vi "wechatDetectCoffeeModel.vi"() -> (0 "Model":string, 1 "ProtoTxt":string)   [LabVIEW 2020]
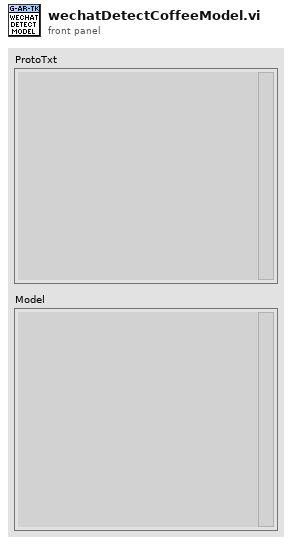
[diagram p1: front panel]
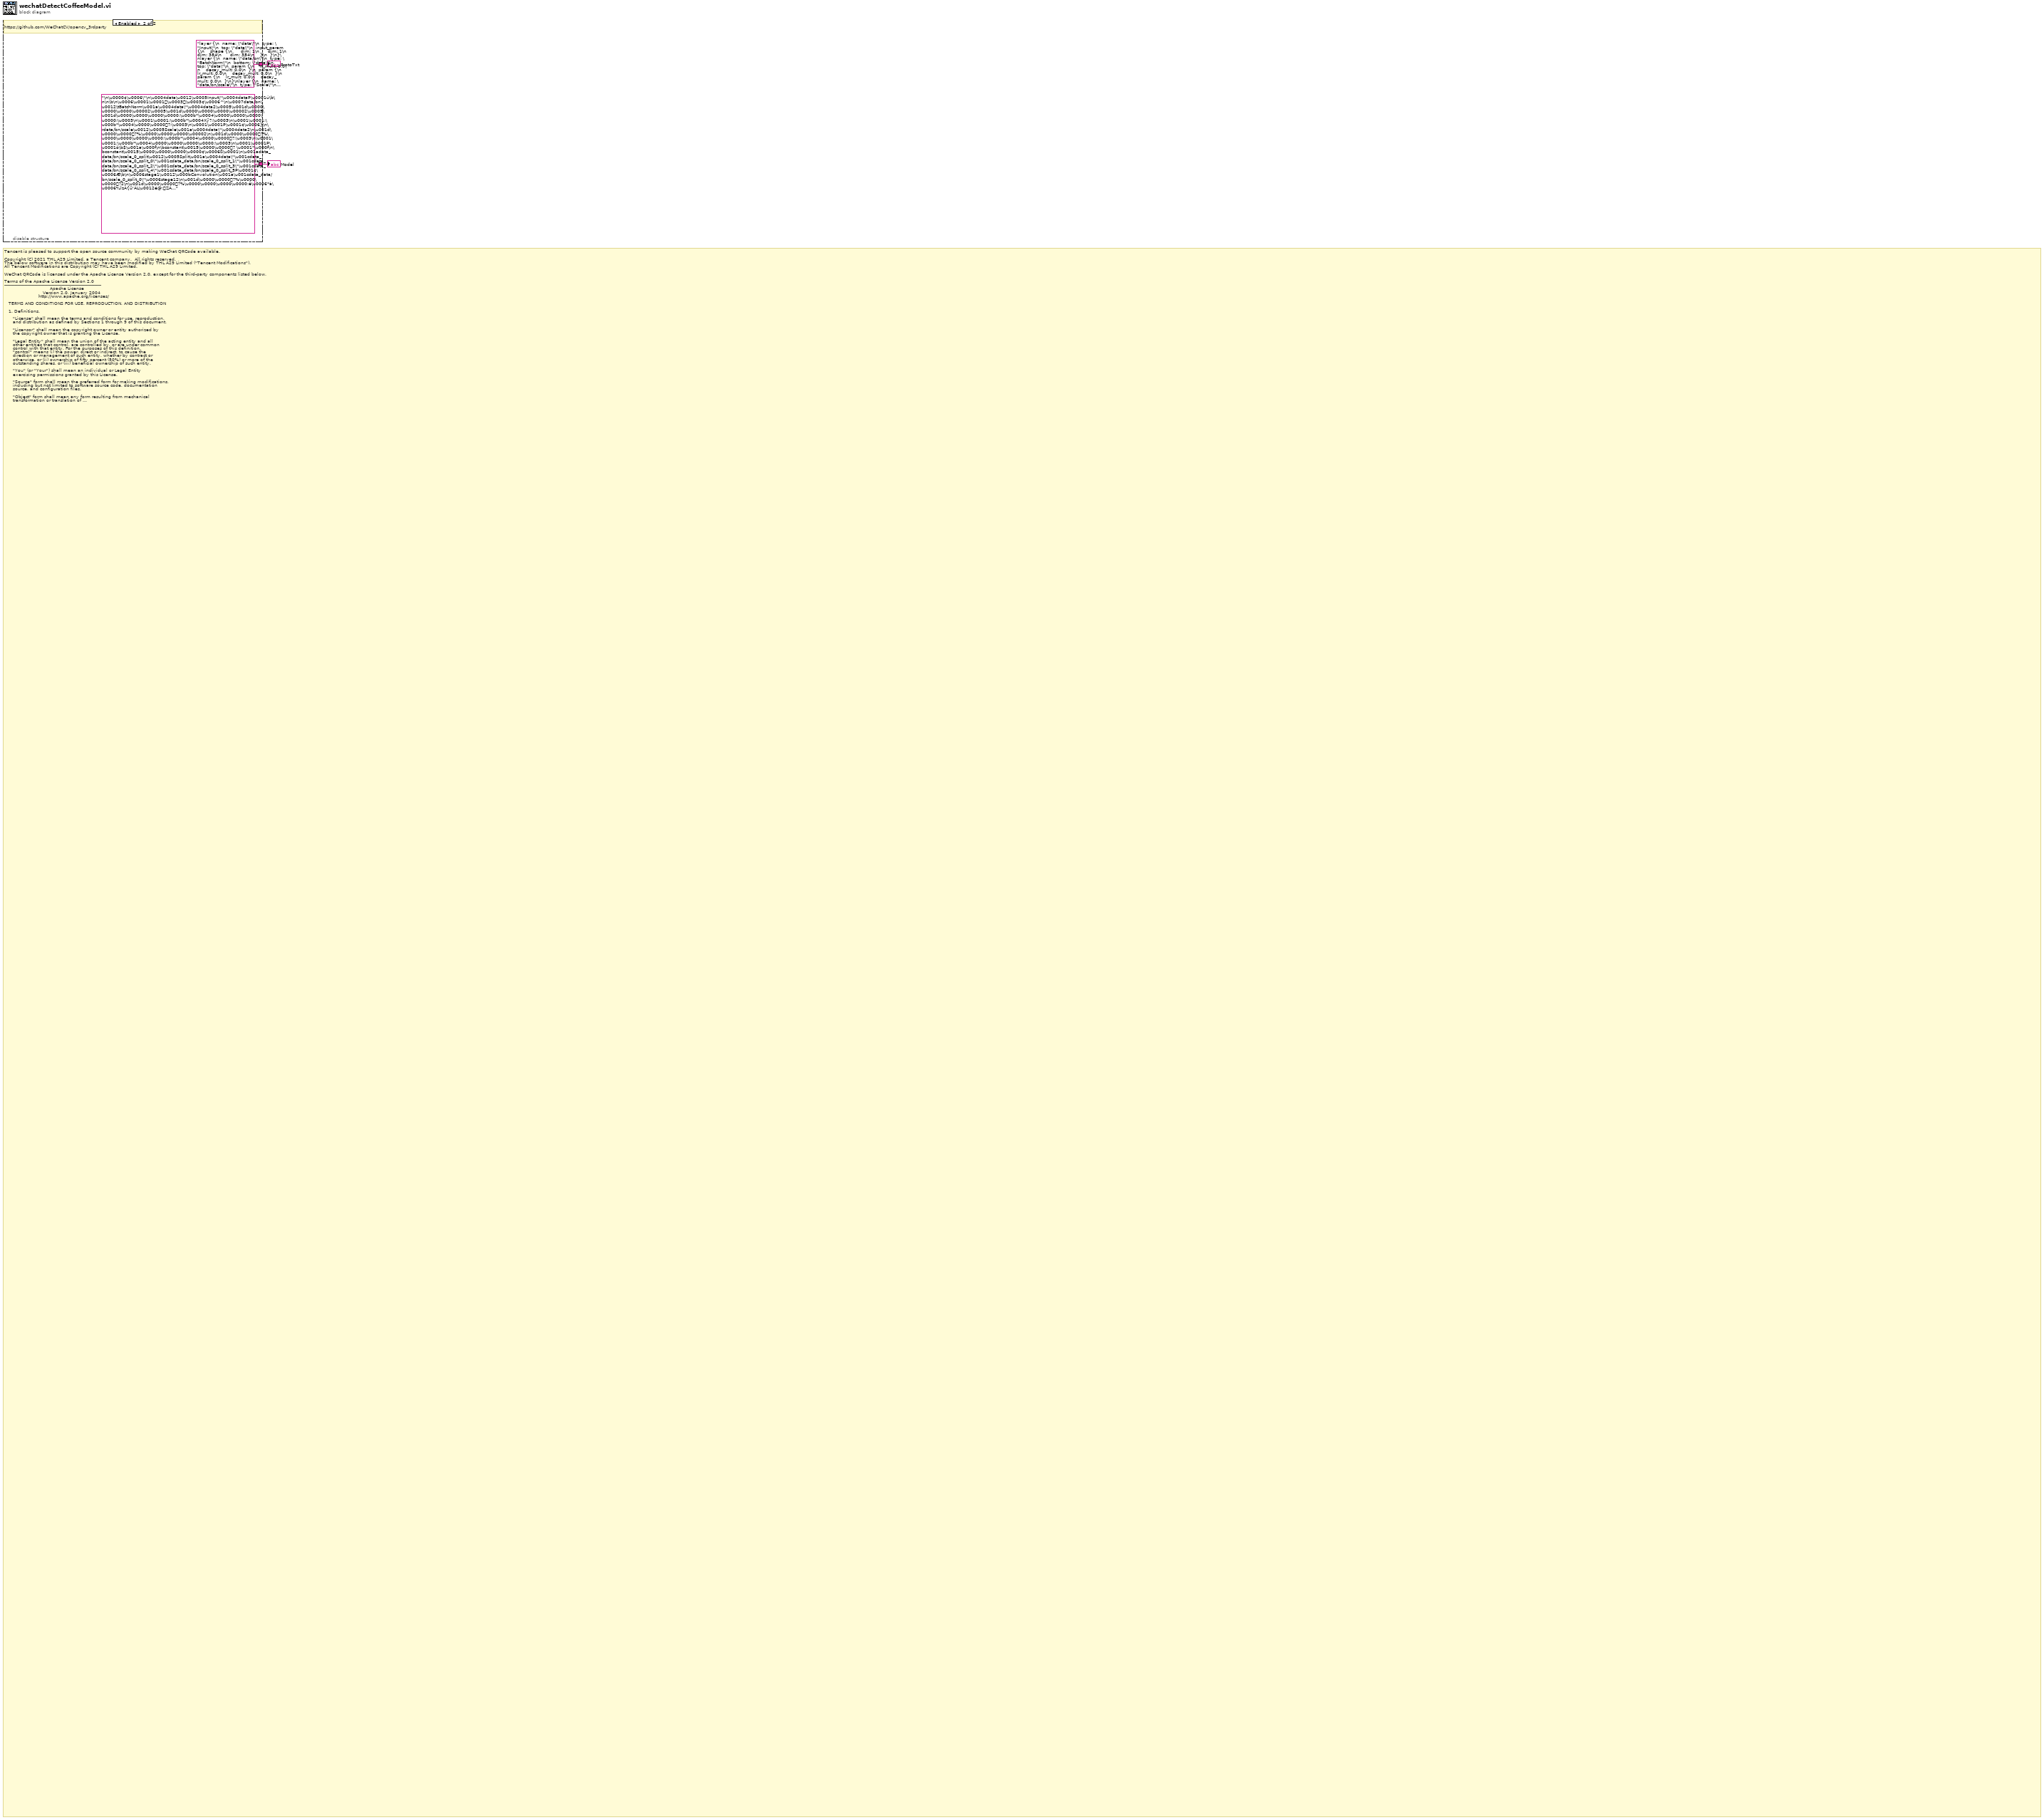
[diagram p0: block diagram]
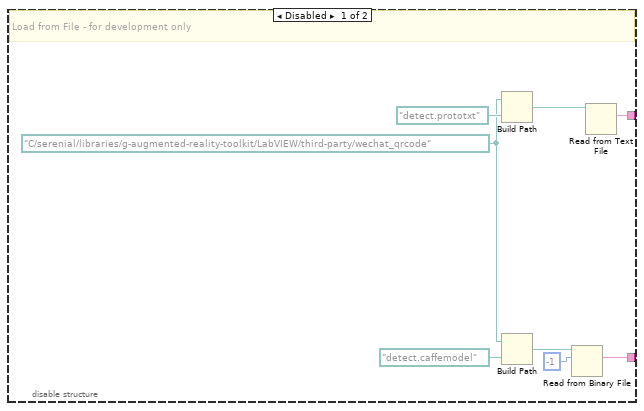
[diagram p2: hidden frame]
diagram:
  # "Tencent is pleased to support the open source community by making WeChat QRCode available.\n\nCopyright (C) 2021 THL A29 Limited, a Tencent company.  All rights reserved.\nThe below software in this distribution may have been modified by THL A29 Limited (\"Tencent Modifications\").\nAll Tencent Modifications are Copyright (C) THL A29 Limited.\n\nWeChat QRCode is licensed under the Apache License Version 2.0, except for the third-party components listed below.\n\nTerms of the Apache License Version 2.0\n--------------------------------------------------------------------\n                                Apache License\n                           Version 2.0, January 2004\n                        http://www.apache.org/licenses/\n\n   TERMS AND CONDITIONS FOR USE, REPRODUCTION, AND DISTRIBUTION\n\n   1. Definitions.\n\n      \"License\" shall mean the terms and conditions for use, reproduction,\n      and distribution as defined by Sections 1 through 9 of this document.\n\n      \"Licensor\" shall mean the copyright owner or entity authorized by\n      the copyright owner that is granting the License.\n\n      \"Legal Entity\" shall mean the union of the acting entity and all\n      other entities that control, are controlled by, or are under common\n      control with that entity. For the purposes of this definition,\n      \"control\" means (i) the power, direct or indirect, to cause the\n      direction or management of such entity, whether by contract or\n      otherwise, or (ii) ownership of fifty percent (50%) or more of the\n      outstanding shares, or (iii) beneficial ownership of such entity.\n\n      \"You\" (or \"Your\") shall mean an individual or Legal Entity\n      exercising permissions granted by this License.\n\n      \"Source\" form shall mean the preferred form for making modifications,\n      including but not limited to software source code, documentation\n      source, and configuration files.\n\n      \"Object\" form shall mean any form resulting from mechanical\n      transformation or translation of a Source form, including but\n      not limited to compiled object code, generated documentation,\n      and conversions to other media types.\n\n      \"Work\" shall mean the work of authorship, whether in Source or\n      Object form, made available under the License, as indicated by a\n      copyright notice that is included in or attached to the work\n      (an example is provided in the Appendix below).\n\n      \"Derivative Works\" shall mean any work, whether in Source or Object\n      form, that is based on (or derived from) the Work and for which the\n      editorial revisions, annotations, elaborations, or other modifications\n      represent, as a whole, an original work of authorship. For the purposes\n      of this License, Derivative Works shall not include works that remain\n      separable from, or merely link (or bind by name) to the interfaces of,\n      the Work and Derivative Works thereof.\n\n      \"Contribution\" shall mean any work of authorship, including\n      the original version of the Work and any modifications or additions\n      to that Work or Derivative Works thereof, that is intentionally\n      submitted to Licensor for inclusion in the Work by the copyright owner\n      or by an individual or Legal Entity authorized to submit on behalf of\n      the copyright owner. For the purposes of this definition, \"submitted\"\n      means any form of electronic, verbal, or written communication sent\n      to the Licensor or its representatives, including but not limited to\n      communication on electronic mailing lists, source code control systems,\n      and issue tracking systems that are managed by, or on behalf of, the\n      Licensor for the purpose of discussing and improving the Work, but\n      excluding communication that is conspicuously marked or otherwise\n      designated in writing by the copyright owner as \"Not a Contribution.\"\n\n      \"Contributor\" shall mean Licensor and any individual or Legal Entity\n      on behalf of whom a Contribution has been received by Licensor and\n      subsequently incorporated within the Work.\n\n   2. Grant of Copyright License. Subject to the terms and conditions of\n      this License, each Contributor hereby grants to You a perpetual,\n      worldwide, non-exclusive, no-charge, royalty-free, irrevocable\n      copyright license to reproduce, prepare Derivative Works of,\n      publicly display, publicly perform, sublicense, and distribute the\n      Work and such Derivative Works in Source or Object form.\n\n   3. Grant of Patent License. Subject to the terms and conditions of\n      this License, each Contributor hereby grants to You a perpetual,\n      worldwide, non-exclusive, no-charge, royalty-free, irrevocable\n      (except as stated in this section) patent license to make, have made,\n      use, offer to sell, sell, import, and otherwise transfer the Work,\n      where such license applies only to those patent claims licensable\n      by such Contributor that are necessarily infringed by their\n      Contribution(s) alone or by combination of their Contribution(s)\n      with the Work to which such Contribution(s) was submitted. If You\n      institute patent litigation against any entity (including a\n      cross-claim or counterclaim in a lawsuit) alleging that the Work\n      or a Contribution incorporated within the Work constitutes direct\n      or contributory patent infringement, then any patent licenses\n      granted to You under this License for that Work shall terminate\n      as of the date such litigation is filed.\n\n   4. Redistribution. You may reproduce and distribute copies of the\n      Work or Derivative Works thereof in any medium, with or without\n      modifications, and in Source or Object form, provided that You\n      meet the following conditions:\n\n      (a) You must give any other recipients of the Work or\n          Derivative Works a copy of this License; and\n\n      (b) You must cause any modified files to carry prominent notices\n          stating that You changed the files; and\n\n      (c) You must retain, in the Source form of any Derivative Works\n          that You distribute, all copyright, patent, trademark, and\n          attribution notices from the Source form of the Work,\n          excluding those notices that do not pertain to any part of\n          the Derivative Works; and\n\n      (d) If the Work includes a \"NOTICE\" text file as part of its\n          distribution, then any Derivative Works that You distribute must\n          include a readable copy of the attribution notices contained\n          within such NOTICE file, excluding those notices that do not\n          pertain to any part of the Derivative Works, in at least one\n          of the following places: within a NOTICE text file distributed\n          as part of the Derivative Works; within the Source form or\n          documentation, if provided along with the Derivative Works; or,\n          within a display generated by the Derivative Works, if and\n          wherever such third-party notices normally appear. The contents\n          of the NOTICE file are for informational purposes only and\n          do not modify the License. You may add Your own attribution\n          notices within Derivative Works that You distribute, alongside\n          or as an addendum to the NOTICE text from the Work, provided\n          that such additional attribution notices cannot be construed\n          as modifying the License.\n\n      You may add Your own copyright statement to Your modifications and\n      may provide additional or different license terms and conditions\n      for use, reproduction, or distribution of Your modifications, or\n      for any such Derivative Works as a whole, provided Your use,\n      reproduction, and distribution of the Work otherwise complies with\n      the conditions stated in this License.\n\n   5. Submission of Contributions. Unless You explicitly state otherwise,\n      any Contribution intentionally submitted for inclusion in the Work\n      by You to the Licensor shall be under the terms and conditions of\n      this License, without any additional terms or conditions.\n      Notwithstanding the above, nothing herein shall supersede or modify\n      the terms of any separate license agreement you may have executed\n      with Licensor regarding such Contributions.\n\n   6. Trademarks. This License does not grant permission to use the trade\n      names, trademarks, service marks, or product names of the Licensor,\n      except as required for reasonable and customary use in describing the\n      origin of the Work and reproducing the content of the NOTICE file.\n\n   7. Disclaimer of Warranty. Unless required by applicable law or\n      agreed to in writing, Licensor provides the Work (and each\n      Contributor provides its Contributions) on an \"AS IS\" BASIS,\n      WITHOUT WARRANTIES OR CONDITIONS OF ANY KIND, either express or\n      implied, including, without limitation, any warranties or conditions\n      of TITLE, NON-INFRINGEMENT, MERCHANTABILITY, or FITNESS FOR A\n      PARTICULAR PURPOSE. You are solely responsible for determining the\n      appropriateness of using or redistributing the Work and assume any\n      risks associated with Your exercise of permissions under this License.\n\n   8. Limitation of Liability. In no event and under no legal theory,\n      whether in tort (including negligence), contract, or otherwise,\n      unless required by applicable law (such as deliberate and grossly\n      negligent acts) or agreed to in writing, shall any Contributor be\n      liable to You for damages, including any direct, indirect, special,\n      incidental, or consequential damages of any character arising as a\n      result of this License or out of the use or inability to use the\n      Work (including but not limited to damages for loss of goodwill,\n      work stoppage, computer failure or malfunction, or any and all\n      other commercial damages or losses), even if such Contributor\n      has been advised of the possibility of such damages.\n\n   9. Accepting Warranty or Additional Liability. While redistributing\n      the Work or Derivative Works thereof, You may choose to offer,\n      and charge a fee for, acceptance of support, warranty, indemnity,\n      or other liability obligations and/or rights consistent with this\n      License. However, in accepting such obligations, You may act only\n      on Your own behalf and on Your sole responsibility, not on behalf\n      of any other Contributor, and only if You agree to indemnify,\n      defend, and hold each Contributor harmless for any liability\n      incurred by, or claims asserted against, such Contributor by reason\n      of your accepting any such warranty or additional liability.\n\nEND OF TERMS AND CONDITIONS\n\n\n\nOther dependencies and licenses:\n\nOpen Source Software Licensed under the Apache License Version 2.0:\n--------------------------------------------------------------------\n1. zxing\nCopyright (c) zxing authors and contributors\nPlease note this software may have been modified by Tencent.\n\nTerms of the Apache License Version 2.0:\n--------------------------------------------------------------------\nApache License\n\nVersion 2.0, January 2004\n\nhttp://www.apache.org/licenses/\n\nTERMS AND CONDITIONS FOR USE, REPRODUCTION, AND DISTRIBUTION\n\n1. Definitions.\n\n\"License\" shall mean the terms and conditions for use, reproduction, and distribution as defined by Sections 1 through 9 of this document.\n\n\"Licensor\" shall mean the copyright owner or entity authorized by the copyright owner that is granting the License.\n\n\"Legal Entity\" shall mean the union of the acting entity and all other entities that control, are controlled by, or are under common control with that entity. For the purposes of this definition, \"control\" means (i) the power, direct or indirect, to cause the direction or management of such entity, whether by contract or otherwise, or (ii) ownership of fifty percent (50%) or more of the outstanding shares, or (iii) beneficial ownership of such entity.\n\n\"You\" (or \"Your\") shall mean an individual or Legal Entity exercising permissions granted by this License.\n\n\"Source\" form shall mean the preferred form for making modifications, including but not limited to software source code, documentation source, and configuration files.\n\n\"Object\" form shall mean any form resulting from mechanical transformation or translation of a Source form, including but not limited to compiled object code, generated documentation, and conversions to other media types.\n\n\"Work\" shall mean the work of authorship, whether in Source or Object form, made available under the License, as indicated by a copyright notice that is included in or attached to the work (an example is provided in the Appendix below).\n\n\"Derivative Works\" shall mean any work, whether in Source or Object form, that is based on (or derived from) the Work and for which the editorial revisions, annotations, elaborations, or other modifications represent, as a whole, an original work of authorship. For the purposes of this License, Derivative Works shall not include works that remain separable from, or merely link (or bind by name) to the interfaces of, the Work and Derivative Works thereof.\n\n\"Contribution\" shall mean any work of authorship, including the original version of the Work and any modifications or additions to that Work or Derivative Works thereof, that is intentionally submitted to Licensor for inclusion in the Work by the copyright owner or by an individual or Legal Entity authorized to submit on behalf of the copyright owner. For the purposes of this definition, \"submitted\" means any form of electronic, verbal, or written communication sent to the Licensor or its representatives, including but not limited to communication on electronic mailing lists, source code control systems, and issue tracking systems that are managed by, or on behalf of, the Licensor for the purpose of discussing and improving the Work, but excluding communication that is conspicuously marked or otherwise designated in writing by the copyright owner as \"Not a Contribution.\"\n\n\"Contributor\" shall mean Licensor and any individual or Legal Entity on behalf of whom a Contribution has been received by Licensor and subsequently incorporated within the Work.\n\n2. Grant of Copyright License. Subject to the terms and conditions of this License, each Contributor hereby grants to You a perpetual, worldwide, non-exclusive, no-charge, royalty-free, irrevocable copyright license to reproduce, prepare Derivative Works of, publicly display, publicly perform, sublicense, and distribute the Work and such Derivative Works in Source or Object form.\n\n3. Grant of Patent License. Subject to the terms and conditions of this License, each Contributor hereby grants to You a perpetual, worldwide, non-exclusive, no-charge, royalty-free, irrevocable (except as stated in this section) patent license to make, have made, use, offer to sell, sell, import, and otherwise transfer the Work, where such license applies only to those patent claims licensable by such Contributor that are necessarily infringed by their Contribution(s) alone or by combination of their Contribution(s) with the Work to which such Contribution(s) was submitted. If You institute patent litigation against any entity (including a cross-claim or counterclaim in a lawsuit) alleging that the Work or a Contribution incorporated within the Work constitutes direct or contributory patent infringement, then any patent licenses granted to You under this License for that Work shall terminate as of the date such litigation is filed.\n\n4. Redistribution. You may reproduce and distribute copies of the Work or Derivative Works thereof in any medium, with or without modifications, and in Source or Object form, provided that You meet the following conditions:\n\nYou must give any other recipients of the Work or Derivative Works a copy of this License; and\nYou must cause any modified files to carry prominent notices stating that You changed the files; and\nYou must retain, in the Source form of any Derivative Works that You distribute, all copyright, patent, trademark, and attribution notices from the Source form of the Work, excluding those notices that do not pertain to any part of the Derivative Works; and\nIf the Work includes a \"NOTICE\" text file as part of its distribution, then any Derivative Works that You distribute must include a readable copy of the attribution notices contained within such NOTICE file, excluding those notices that do not pertain to any part of the Derivative Works, in at least one of the following places: within a NOTICE text file distributed as part of the Derivative Works; within the Source form or documentation, if provided along with the Derivative Works; or, within a display generated by the Derivative Works, if and wherever such third-party notices normally appear. The contents of the NOTICE file are for informational purposes only and do not modify the License. You may add Your own attribution notices within Derivative Works that You distribute, alongside or as an addendum to the NOTICE text from the Work, provided that such additional attribution notices cannot be construed as modifying the License.\n\nYou may add Your own copyright statement to Your modifications and may provide additional or different license terms and conditions for use, reproduction, or distribution of Your modifications, or for any such Derivative Works as a whole, provided Your use, reproduction, and distribution of the Work otherwise complies with the conditions stated in this License.\n\n5. Submission of Contributions. Unless You explicitly state otherwise, any Contribution intentionally submitted for inclusion in the Work by You to the Licensor shall be under the terms and conditions of this License, without any additional terms or conditions. Notwithstanding the above, nothing herein shall supersede or modify the terms of any separate license agreement you may have executed with Licensor regarding such Contributions.\n\n6. Trademarks. This License does not grant permission to use the trade names, trademarks, service marks, or product names of the Licensor, except as required for reasonable and customary use in describing the origin of the Work and reproducing the content of the NOTICE file.\n\n7. Disclaimer of Warranty. Unless required by applicable law or agreed to in writing, Licensor provides the Work (and each Contributor provides its Contributions) on an \"AS IS\" BASIS, WITHOUT WARRANTIES OR CONDITIONS OF ANY KIND, either express or implied, including, without limitation, any warranties or conditions of TITLE, NON-INFRINGEMENT, MERCHANTABILITY, or FITNESS FOR A PARTICULAR PURPOSE. You are solely responsible for determining the appropriateness of using or redistributing the Work and assume any risks associated with Your exercise of permissions under this License.\n\n8. Limitation of Liability. In no event and under no legal theory, whether in tort (including negligence), contract, or otherwise, unless required by applicable law (such as deliberate and grossly negligent acts) or agreed to in writing, shall any Contributor be liable to You for damages, including any direct, indirect, special, incidental, or consequential damages of any character arising as a result of this License or out of the use or inability to use the Work (including but not limited to damages for loss of goodwill, work stoppage, computer failure or malfunction, or any and all other commercial damages or losses), even if such Contributor has been advised of the possibility of such damages.\n\n9. Accepting Warranty or Additional Liability. While redistributing the Work or Derivative Works thereof, You may choose to offer, and charge a fee for, acceptance of support, warranty, indemnity, or other liability obligations and/or rights consistent with this License. However, in accepting such obligations, You may act only on Your own behalf and on Your sole responsibility, not on behalf of any other Contributor, and only if You agree to indemnify, defend, and hold each Contributor harmless for any liability incurred by, or claims asserted against, such Contributor by reason of your accepting any such warranty or additional liability.\n\nEND OF TERMS AND CONDITIONS"
  n1 = disable-structure shown="Enabled" {
    disable-tunnel: [w5 "\n\u0000¢\u0006\"\n\u0004data\u0012\u0005Input\"\u0004dataP\u0001ú\b\n\n\b\n\u0006\u0001\u0001\u0003\u0003¢\u0006^\n\u0007data/bn\u0012\tBatchNorm\u001a\u0004data\"\u0004data2\u0005\u001d\u0000\u0000\u0000\u00002\u0005\u001d\u0000\u0000\u0000\u00002\u0005\u001d\u0000\u0000\u0000\u0000:\u000b*\u0004\u0000\u0000\u0000\u0000:\u0003\n\u0001\u0001:\u000b*\u0004Xÿ?:\u0003\n\u0001\u0001:\u000b*\u0004\u0000\u0000?:\u0003\n\u0001\u0001P\u0001¢\u0006}\n\rdata/bn/scale\u0012\u0005Scale\u001a\u0004data\"\u0004data2\n\u001d\u0000\u0000?%\u0000\u0000\u0000\u00002\n\u001d\u0000\u0000?%\u0000\u0000\u0000\u0000:\u000b*\u0004\u0000\u0000?:\u0003\n\u0001\u0001:\u000b*\u0004\u0000\u0000\u0000\u0000:\u0003\n\u0001\u0001P\u0001ò\b$\u001a\u000f\n\bconstant\u0015\u0000\u0000? \u0001*\u000f\n\bconstant\u0015\u0000\u0000\u0000\u0000¢\u0006ß\u0001\n\u001adata_data/bn/scale_0_split\u0012\u0005Split\u001a\u0004data\"\u001cdata_data/bn/scale_0_split_0\"\u001cdata_data/bn/scale_0_split_1\"\u001cdata_data/bn/scale_0_split_2\"\u001cdata_data/bn/scale_0_split_3\"\u001cdata_data/bn/scale_0_split_4\"\u001cdata_data/bn/scale_0_split_5P\u0001¢\u0006Æ\b\n\u0006stage1\u0012\u000bConvolution\u001a\u001cdata_data/bn/scale_0_split_0\"\u0006stage12\n\u001d\u0000\u0000?%\u0000\u0000?2\n\u001d\u0000\u0000?%\u0000\u0000\u0000\u0000:ë\u0006*à\u0006¼lzÀ{ü'ÁL\u0012é@:ZÁ..." ("Model")] -> w2
    disable-tunnel: [w3 "layer {\n  name: \"data\"\n  type: \"Input\"\n  top: \"data\"\n  input_param {\n    shape {\n      dim: 1\n      dim: 1\n      dim: 384\n      dim: 384\n    }\n  }\n}\nlayer {\n  name: \"data/bn\"\n  type: \"BatchNorm\"\n  bottom: \"data\"\n  top: \"data\"\n  param {\n    lr_mult: 0.0\n    decay_mult: 0.0\n  }\n  param {\n    lr_mult: 0.0\n    decay_mult: 0.0\n  }\n  param {\n    lr_mult: 0.0\n    decay_mult: 0.0\n  }\n}\nlayer {\n  name: \"data/bn/scale\"\n  type: \"Scale\"\n  bottom: \"data\"\n  top: \"data\"\n  param {\n    lr_mult: 1.0\n    decay_mult: 0.0\n  }\n  param {\n    lr_mult: 1.0\n    decay_mult: 0.0\n  }\n  scale_param {\n    filler {\n      type: \"constant\"\n      value: 1.0\n    }\n    bias_term: true\n    bias_filler {\n      type: \"constant\"\n      value: 0.0\n    }\n  }\n}\nlayer {\n  name: \"stage1\"\n  type: \"Convolution\"\n  bottom: \"data\"\n  top: \"stage1\"\n  param {\n    lr_mult: 1.0\n    decay_mult: 1.0\n  }\n  param {\n    lr_mult: 1.0\n    decay_mult: 0.0\n  }\n  convolution_param {\n    num_output: 24\n    bias_term: true\n    pad: 1\n    kernel_size: 3\n    group: 1\n    stride: 2\n    weight_filler {\n      type: \"msra\"\n    }\n    dilation: 1\n  }\n}\nlayer {\n  name: \"stage1/bn\"\n  type: \"BatchNorm\"\n  bottom: \"stage1\"\n  top: \"stage1\"\n  param {\n    lr_mult: 0.0\n    decay_mult: 0.0\n  }\n  param {\n    lr_mult: 0.0\n    decay_mult: 0.0\n  }\n  param {\n    lr_mult: 0.0\n    decay_mult: 0.0\n  }\n}\nlayer {\n  name: \"stage1/bn/scale\"\n  type: \"Scale\"\n  bottom: \"stage1\"\n  top: \"stage1\"\n  param {\n    lr_mult: 1.0\n    decay_mult: 0.0\n  }\n  param {\n    lr_mult: 1.0\n    decay_mult: 0.0\n  }\n  scale_param {\n    filler {\n      type: \"constant\"\n      value: 1.0\n    }\n    bias_term: true\n    bias_filler {\n      type: \"constant\"\n      value: 0.0\n    }\n  }\n}\nlayer {\n  name: \"stage1/relu\"\n  type: \"ReLU\"\n  bottom: \"stage1\"\n  top: \"stage1\"\n}\nlayer {\n  name: \"stage2\"\n  type: \"Pooling\"\n  bottom: \"stage1\"\n  top: \"stage2\"\n  pooling_param {\n    pool: MAX\n    kernel_size: 3\n    stride: 2\n    pad: 0\n  }\n}\nlayer {\n  name: \"stage3_1/conv1\"\n  type: \"Convolution\"\n  bottom: \"stage2\"\n  top: \"stage3_1/conv1\"\n  param {\n    lr_mult: 1.0\n    decay_mult: 1.0\n  }\n  convolution_param {\n    num_output: 16\n    pad: 0\n    kernel_size: 1\n    group: 1\n    stride: 1\n    weight_filler {\n      type: \"msra\"\n    }\n    dilation: 1\n  }\n}\nlayer {\n  name: \"stage3_1/conv1/relu\"\n  type: \"ReLU\"\n  bottom: \"stage3_1/conv1\"\n  top: \"stage3_1/conv1\"\n}\nlayer {\n  name: \"stage3_1/conv2\"\n  type: \"Convolution\"\n  bottom: \"stage3_1/conv1\"\n  top: \"stage3_1/conv2\"\n  param {\n    lr_mult: 1.0\n    decay_mult: 1.0\n  }\n  convolution_param {\n    num_output: 16\n    pad: 1\n    kernel_size: 3\n    group: 16\n    stride: 2\n    weight_filler {\n      type: \"msra\"\n    }\n    dilation: 1\n  }\n}\nlayer {\n  name: \"stage3_1/conv3\"\n  type: \"Convolution\"\n  bottom: \"stage3_1/conv2\"\n  top: \"stage3_1/conv3\"\n  param {\n    lr_mult: 1.0\n    decay_mult: 1.0\n  }\n  convolution_param {\n    num_output: 64\n    pad: 0\n    kernel_size: 1\n    group: 1\n    stride: 1\n    weight_filler {\n      type: \"msra\"\n    }\n    dilation: 1\n  }\n}\nlayer {\n  name: \"stage3_1/relu\"\n  type: \"ReLU\"\n  bottom: \"stage3_1/conv3\"\n  top: \"stage3_1/conv3\"\n}\nlayer {\n  name: \"stage3_2/conv1\"\n  type: \"Convolution\"\n  bottom: \"stage3_1/conv3\"\n  top: \"stage3_2/conv1\"\n  param {\n    lr_mult: 1.0\n    decay_mult: 1.0\n  }\n  convolution_param {\n    num_output: 16\n    pad: 0\n    kernel_size: 1\n    group: 1\n    stride: 1\n    weight_filler {\n      type: \"msra\"\n    }\n    dilation: 1\n  }\n}\nlayer {\n  name: \"stage3_2/conv1/relu\"\n  type: \"ReLU\"\n  bottom: \"stage3_2/conv1\"\n  top: \"stage3_2/conv1\"\n}\nlayer {\n  name: \"stage3_2/conv2\"\n  type: \"Convolution\"\n  bottom: \"stage3_2/conv1\"\n  top: \"stage3_2/conv2\"\n  param {\n    lr_mult: 1.0\n    decay_mult: 1.0\n  }\n  convolution_param {\n    num_output: 16\n    pad: 1\n    kernel_size: 3\n    group: 16\n    stride: 1\n    weight_filler {\n      type: \"msra\"\n    }\n    dilation: 1\n  }\n}\nlayer {\n  name: \"stage3_2/conv3\"\n  type: \"Convolution\"\n  bottom: \"stage3_2/conv2\"\n  top: \"stage3_2/conv3\"\n  param {\n    lr_mult: 1.0\n    decay_mult: 1.0\n  }\n  convolution_param {\n    num_output: 64\n    pad: 0\n    kernel_size: 1\n    group: 1\n    stride: 1\n    weight_filler {\n      type: \"msra\"\n    }\n    dilation: 1\n  }\n}\nlayer {\n  name: \"stage3_2/sum\"\n  type: \"Eltwise\"\n  bottom: \"stage3_1/conv3\"\n  bottom: \"stage3_2/conv3\"\n  top: \"stage3_2/sum\"\n  eltwise_param {\n    operation: SUM\n  }\n}\nlayer {\n  name: \"stage3_2/relu\"\n  type: \"ReLU\"\n  bottom: \"stage3_2/sum\"\n  top: \"stage3_2/sum\"\n}\nlayer {\n  name: \"stage3_3/conv1\"\n  type: \"Convolution\"\n  bottom: \"stage3_2/sum\"\n  top: \"stage3_3/conv1\"\n  param {\n    lr_mult: 1.0\n    decay_mult: 1.0\n  }\n  convolution_param {\n    num_output: 16\n    pad: 0\n    kernel_size: 1\n    group: 1\n    stride: 1\n    weight_filler {\n      type: \"msra\"\n    }\n    dilation: 1\n  }\n}\nlayer {\n  name: \"stage3_3/conv1/relu\"\n  type: \"ReLU\"\n  bottom: \"stage3_3/conv1\"\n  top: \"stage3_3/conv1\"\n}\nlayer {\n  name: \"stage3_3/conv2\"\n  type: \"Convolution\"\n  bottom: \"stage3_3/conv1\"\n  top: \"stage3_3/conv2\"\n  param {\n    lr_mult: 1.0\n    decay_mult: 1.0\n  }\n  convolution_param {\n    num_output: 16\n    pad: 1\n    kernel_size: 3\n    group: 16\n    stride: 1\n    weight_filler {\n      type: \"msra\"\n    }\n    dilation: 1\n  }\n}\nlayer {\n  name: \"stage3_3/conv3\"\n  type: \"Convolution\"\n  bottom: \"stage3_3/conv2\"\n  top: \"stage3_3/conv3\"\n  param {\n    lr_mult: 1.0\n    decay_mult: 1.0\n  }\n  convolution_param {\n    num_output: 64\n    pad: 0\n    kernel_size: 1\n    group: 1\n    stride: 1\n    weight_filler {\n      type: \"msra\"\n    }\n    dilation: 1\n  }\n}\nlayer {\n  name: \"stage3_3/sum\"\n  type: \"Eltwise\"\n  bottom: \"stage3_2/sum\"\n  bottom: \"stage3_3/conv3\"\n  top: \"stage3_3/sum\"\n  eltwise_param {\n    operation: SUM\n  }\n}\nlayer {\n  name: \"stage3_3/relu\"\n  type: \"ReLU\"\n  bottom: \"stage3_3/sum\"\n  top: \"stage3_3/sum\"\n}\nlayer {\n  name: \"stage3_4/conv1\"\n  type: \"Convolution\"\n  bottom: \"stage3_3/sum\"\n  top: \"stage3_4/conv1\"\n  param {\n    lr_mult: 1.0\n    decay_mult: 1.0\n  }\n  convolution_param {\n    num_output: 16\n    pad: 0\n    kernel_size: 1\n    group: 1\n    stride: 1\n    weight_filler {\n      type: \"msra\"\n    }\n    dilation: 1\n  }\n}\nlayer {\n  name: \"stage3_4/conv1/relu\"\n  type: \"ReLU\"\n  bottom: \"stage3_4/conv1\"\n  top: \"stage3_4/conv1\"\n}\nlayer {\n  name: \"stage3_4/conv2\"\n  type: \"Convolution\"\n  bottom: \"stage3_4/conv1\"\n  top: \"stage3_4/conv2\"\n  param {\n    lr_mult: 1.0\n    decay_mult: 1.0\n  }\n  convolution_param {\n    num_output: 16\n    pad: 1\n    kernel_size: 3\n    group: 16\n    stride: 1\n    weight_filler {\n      type: \"msra\"\n    }\n    dilation: 1\n  }\n}\nlayer {\n  name: \"stage3_4/conv3\"\n  type: \"Convolution\"\n  bottom: \"stage3_4/conv2\"\n  top: \"stage3_4/conv3\"\n  param {\n    lr_mult: 1.0\n    decay_mult: 1.0\n  }\n  convolution_param {\n    num_output: 64\n    pad: 0\n    kernel_size: 1\n    group: 1\n    stride: 1\n    weight_filler {\n      type: \"msra\"\n    }\n    dilation: 1\n  }\n}\nlayer {\n  name: \"stage3_4/sum\"\n  type: \"Eltwise\"\n  bottom: \"stage3_3/sum\"\n  bottom: \"stage3_4/conv3\"\n  top: \"stage3_4/sum\"\n  eltwise_param {\n    operation: SUM\n  }\n}\nlayer {\n  name: \"stage3_4/relu\"\n  type: \"ReLU\"\n  bottom: \"stage3_4/sum\"\n  top: \"stage3_4/sum\"\n}\nlayer {\n  name: \"stage4_1/conv1\"\n  type: \"Convolution\"\n  bottom: \"stage3_4/sum\"\n  top: \"stage4_1/conv1\"\n  param {\n    lr_mult: 1.0\n    decay_mult: 1.0\n  }\n  convolution_param {\n    num_output: 32\n    pad: 0\n    kernel_size: 1\n    group: 1\n    stride: 1\n    weight_filler {\n      type: \"msra\"\n    }\n    dilation: 1\n  }\n}\nlayer {\n  name: \"stage4_1/conv1/relu\"\n  type: \"ReLU\"\n  bottom: \"stage4_1/conv1\"\n  top: \"stage4_1/conv1\"\n}\nlayer {\n  name: \"stage4_1/conv2\"\n  type: \"Convolution\"\n  bottom: \"stage4_1/conv1\"\n  top: \"stage4_1/conv2\"\n  param {\n    lr_mult: 1.0\n    decay_mult: 1.0\n  }\n  convolution_param {\n    num_output: 32\n    pad: 1\n    kernel_size: 3\n    group: 32\n    stride: 2\n    weight_filler {\n      type: \"msra\"\n    }\n    dilation: 1\n  }\n}\nlayer {\n  name: \"stage4_1/conv3\"\n  type: \"Convolution\"\n  bottom: \"stage4_1/conv2\"\n  top: \"stage4_1/conv3\"\n  param {\n    lr_mult: 1.0\n    decay_mult: 1.0\n  }\n  convolution_param {\n    num_output: 128\n    pad: 0\n    kernel_size: 1\n    group: 1\n    stride: 1\n    weight_filler {\n      type: \"msra\"\n    }\n    dilation: 1\n  }\n}\nlayer {\n  name: \"stage4_1/relu\"\n  type: \"ReLU\"\n  bottom: \"stage4_1/conv3\"\n  top: \"stage4_1/conv3\"\n}\nlayer {\n  name: \"stage4_2/conv1\"\n  type: \"Convolution\"\n  bottom: \"stage4_1/conv3\"\n  top: \"stage4_2/conv1\"\n  param {\n    lr_mult: 1.0\n    decay_mult: 1.0\n  }\n  convolution_param {\n    num_output: 32\n    pad: 0\n    kernel_size: 1\n    group: 1\n    stride: 1\n    weight_filler {\n      type: \"msra\"\n    }\n    dilation: 1\n  }\n}\nlayer {\n  name: \"stage4_2/conv1/relu\"\n  type: \"ReLU\"\n  bottom: \"stage4_2/conv1\"\n  top: \"stage4_2/conv1\"\n}\nlayer {\n  name: \"stage4_2/conv2\"\n  type: \"Convolution\"\n  bottom: \"stage4_2/conv1\"\n  top: \"stage4_2/conv2\"\n  param {\n    lr_mult: 1.0\n    decay_mult: 1.0\n  }\n  convolution_param {\n    num_output: 32\n    pad: 1\n    kernel_size: 3\n    group: 32\n    stride: 1\n    weight_filler {\n      type: \"msra\"\n    }\n    dilation: 1\n  }\n}\nlayer {\n  name: \"stage4_2/conv3\"\n  type: \"Convolution\"\n  bottom: \"stage4_2/conv2\"\n  top: \"stage4_2/conv3\"\n  param {\n    lr_mult: 1.0\n    decay_mult: 1.0\n  }\n  convolution_param {\n    num_output: 128\n    pad: 0\n    kernel_size: 1\n    group: 1\n    stride: 1\n    weight_filler {\n      type: \"msra\"\n    }\n    dilation: 1\n  }\n}\nlayer {\n  name: \"stage4_2/sum\"\n  type: \"Eltwise\"\n  bottom: \"stage4_1/conv3\"\n  bottom: \"stage4_2/conv3\"\n  top: \"stage4_2/sum\"\n  eltwise_param {\n    operation: SUM\n  }\n}\nlayer {\n  name: \"stage4_2/relu\"\n  type: \"ReLU\"\n  bottom: \"stage4_2/sum\"\n  top: \"stage4_2/sum\"\n}\nlayer {\n  name: \"stage4_3/conv1\"\n  type: \"Convolution\"\n  bottom: \"stage4_2/sum\"\n  top: \"stage4_3/conv1\"\n  param {\n    lr_mult: 1.0\n    decay_mult: 1.0\n  }\n  convolution_param {\n    num_output: 32\n    pad: 0\n    kernel_size: 1\n    group: 1\n    stride: 1\n    weight_filler {\n      type: \"msra\"\n    }\n    dilation: 1\n  }\n}\nlayer {\n  name: \"stage4_3/conv1/relu\"\n  type: \"ReLU\"\n  bottom: \"stage4_3/conv1\"\n  top: \"stage4_3/conv1\"\n}\nlayer {\n  name: \"stage4_3/conv2\"\n  type: \"Convolution\"\n  bottom: \"stage4_3/conv1\"\n  top: \"stage4_3/conv2\"\n  param {\n    lr_mult: 1.0\n    decay_mult: 1.0\n  }\n  convolution_param {\n    num_output: 32\n    pad: 1\n    kernel_size: 3\n    group: 32\n    stride: 1\n    weight_filler {\n      type: \"msra\"\n    }\n    dilation: 1\n  }\n}\nlayer {\n  name: \"stage4_3/conv3\"\n  type: \"Convolution\"\n  bottom: \"stage4_3/conv2\"\n  top: \"stage4_3/conv3\"\n  param {\n    lr_mult: 1.0\n    decay_mult: 1.0\n  }\n  convolution_param {\n    num_output: 128\n    pad: 0\n    kernel_size: 1\n    group: 1\n    stride: 1\n    weight_filler {\n      type: \"msra\"\n    }\n    dilation: 1\n  }\n}\nlayer {\n  name: \"stage4_3/sum\"\n  type: \"Eltwise\"\n  bottom: \"stage4_2/sum\"\n  bottom: \"stage4_3/conv3\"\n  top: \"stage4_3/sum\"\n  eltwise_param {\n    operation: SUM\n  }\n}\nlayer {\n  name: \"stage4_3/relu\"\n  type: \"ReLU\"\n  bottom: \"stage4_3/sum\"\n  top: \"stage4_3/sum\"\n}\nlayer {\n  name: \"stage4_4/conv1\"\n  type: \"Convolution\"\n  bottom: \"stage4_3/sum\"\n  top: \"stage4_4/conv1\"\n  param {\n    lr_mult: 1.0\n    decay_mult: 1.0\n  }\n  convolution_param {\n    num_output: 32\n    pad: 0\n    kernel_size: 1\n    group: 1\n    stride: 1\n    weight_filler {\n      type: \"msra\"\n    }\n    dilation: 1\n  }\n}\nlayer {\n  name: \"stage4_4/conv1/relu\"\n  type: \"ReLU\"\n  bottom: \"stage4_4/conv1\"\n  top: \"stage4_4/conv1\"\n}\nlayer {\n  name: \"stage4_4/conv2\"\n  type: \"Convolution\"\n  bottom: \"stage4_4/conv1\"\n  top: \"stage4_4/conv2\"\n  param {\n    lr_mult: 1.0\n    decay_mult: 1.0\n  }\n  convolution_param {\n    num_output: 32\n    pad: 1\n    kernel_size: 3\n    group: 32\n    stride: 1\n    weight_filler {\n      type: \"msra\"\n    }\n    dilation: 1\n  }\n}\nlayer {\n  name: \"stage4_4/conv3\"\n  type: \"Convolution\"\n  bottom: \"stage4_4/conv2\"\n  top: \"stage4_4/conv3\"\n  param {\n    lr_mult: 1.0\n    decay_mult: 1.0\n  }\n  convolution_param {\n    num_output: 128\n    pad: 0\n    kernel_size: 1\n    group: 1\n    stride: 1\n    weight_filler {\n      type: \"msra\"\n    }\n    dilation: 1\n  }\n}\nlayer {\n  name: \"stage4_4/sum\"\n  type: \"Eltwise\"\n  bottom: \"stage4_3/sum\"\n  bottom: \"stage4_4/conv3\"\n  top: \"stage4_4/sum\"\n  eltwise_param {\n    operation: SUM\n  }\n}\nlayer {\n  name: \"stage4_4/relu\"\n  type: \"ReLU\"\n  bottom: \"stage4_4/sum\"\n  top: \"stage4_4/sum\"\n}\nlayer {\n  name: \"stage4_5/conv1\"\n  type: \"Convolution\"\n  bottom: \"stage4_4/sum\"\n  top: \"stage4_5/conv1\"\n  param {\n    lr_mult: 1.0\n    decay_mult: 1.0\n  }\n  convolution_param {\n    num_output: 32\n    pad: 0\n    kernel_size: 1\n    group: 1\n    stride: 1\n    weight_filler {\n      type: \"msra\"\n    }\n    dilation: 1\n  }\n}\nlayer {\n  name: \"stage4_5/conv1/relu\"\n  type: \"ReLU\"\n  bottom: \"stage4_5/conv1\"\n  top: \"stage4_5/conv1\"\n}\nlayer {\n  name: \"stage4_5/conv2\"\n  type: \"Convolution\"\n  bottom: \"stage4_5/conv1\"\n  top: \"stage4_5/conv2\"\n  param {\n    lr_mult: 1.0\n    decay_mult: 1.0\n  }\n  convolution_param {\n    num_output: 32\n    pad: 1\n    kernel_size: 3\n    group: 32\n    stride: 1\n    weight_filler {\n      type: \"msra\"\n    }\n    dilation: 1\n  }\n}\nlayer {\n  name: \"stage4_5/conv3\"\n  type: \"Convolution\"\n  bottom: \"stage4_5/conv2\"\n  top: \"stage4_5/conv3\"\n  param {\n    lr_mult: 1.0\n    decay_mult: 1.0\n  }\n  convolution_param {\n    num_output: 128\n    pad: 0\n    kernel_size: 1\n    group: 1\n    stride: 1\n    weight_filler {\n      type: \"msra\"\n    }\n    dilation: 1\n  }\n}\nlayer {\n  name: \"stage4_5/sum\"\n  type: \"Eltwise\"\n  bottom: \"stage4_4/sum\"\n  bottom: \"stage4_5/conv3\"\n  top: \"stage4_5/sum\"\n  eltwise_param {\n    operation: SUM\n  }\n}\nlayer {\n  name: \"stage4_5/relu\"\n  type: \"ReLU\"\n  bottom: \"stage4_5/sum\"\n  top: \"stage4_5/sum\"\n}\nlayer {\n  name: \"stage4_6/conv1\"\n  type: \"Convolution\"\n  bottom: \"stage4_5/sum\"\n  top: \"stage4_6/conv1\"\n  param {\n    lr_mult: 1.0\n    decay_mult: 1.0\n  }\n  convolution_param {\n    num_output: 32\n    pad: 0\n    kernel_size: 1\n    group: 1\n    stride: 1\n    weight_filler {\n      type: \"msra\"\n    }\n    dilation: 1\n  }\n}\nlayer {\n  name: \"stage4_6/conv1/relu\"\n  type: \"ReLU\"\n  bottom: \"stage4_6/conv1\"\n  top: \"stage4_6/conv1\"\n}\nlayer {\n  name: \"stage4_6/conv2\"\n  type: \"Convolution\"\n  bottom: \"stage4_6/conv1\"\n  top: \"stage4_6/conv2\"\n  param {\n    lr_mult: 1.0\n    decay_mult: 1.0\n  }\n  convolution_param {\n    num_output: 32\n    pad: 1\n    kernel_size: 3\n    group: 32\n    stride: 1\n    weight_filler {\n      type: \"msra\"\n    }\n    dilation: 1\n  }\n}\nlayer {\n  name: \"stage4_6/conv3\"\n  type: \"Convolution\"\n  bottom: \"stage4_6/conv2\"\n  top: \"stage4_6/conv3\"\n  param {\n    lr_mult: 1.0\n    decay_mult: 1.0\n  }\n  convolution_param {\n    num_output: 128\n    pad: 0\n    kernel_size: 1\n    group: 1\n    stride: 1\n    weight_filler {\n      type: \"msra\"\n    }\n    dilation: 1\n  }\n}\nlayer {\n  name: \"stage4_6/sum\"\n  type: \"Eltwise\"\n  bottom: \"stage4_5/sum\"\n  bottom: \"stage4_6/conv3\"\n  top: \"stage4_6/sum\"\n  eltwise_param {\n    operation: SUM\n  }\n}\nlayer {\n  name: \"stage4_6/relu\"\n  type: \"ReLU\"\n  bottom: \"stage4_6/sum\"\n  top: \"stage4_6/sum\"\n}\nlayer {\n  name: \"stage4_7/conv1\"\n  type: \"Convolution\"\n  bottom: \"stage4_6/sum\"\n  top: \"stage4_7/conv1\"\n  param {\n    lr_mult: 1.0\n    decay_mult: 1.0\n  }\n  convolution_param {\n    num_output: 32\n    pad: 0\n    kernel_size: 1\n    group: 1\n    stride: 1\n    weight_filler {\n      type: \"msra\"\n    }\n    dilation: 1\n  }\n}\nlayer {\n  name: \"stage4_7/conv1/relu\"\n  type: \"ReLU\"\n  bottom: \"stage4_7/conv1\"\n  top: \"stage4_7/conv1\"\n}\nlayer {\n  name: \"stage4_7/conv2\"\n  type: \"Convolution\"\n  bottom: \"stage4_7/conv1\"\n  top: \"stage4_7/conv2\"\n  param {\n    lr_mult: 1.0\n    decay_mult: 1.0\n  }\n  convolution_param {\n    num_output: 32\n    pad: 1\n    kernel_size: 3\n    group: 32\n    stride: 1\n    weight_filler {\n      type: \"msra\"\n    }\n    dilation: 1\n  }\n}\nlayer {\n  name: \"stage4_7/conv3\"\n  type: \"Convolution\"\n  bottom: \"stage4_7/conv2\"\n  top: \"stage4_7/conv3\"\n  param {\n    lr_mult: 1.0\n    decay_mult: 1.0\n  }\n  convolution_param {\n    num_output: 128\n    pad: 0\n    kernel_size: 1\n    group: 1\n    stride: 1\n    weight_filler {\n      type: \"msra\"\n    }\n    dilation: 1\n  }\n}\nlayer {\n  name: \"stage4_7/sum\"\n  type: \"Eltwise\"\n  bottom: \"stage4_6/sum\"\n  bottom: \"stage4_7/conv3\"\n  top: \"stage4_7/sum\"\n  eltwise_param {\n    operation: SUM\n  }\n}\nlayer {\n  name: \"stage4_7/relu\"\n  type: \"ReLU\"\n  bottom: \"stage4_7/sum\"\n  top: \"stage4_7/sum\"\n}\nlayer {\n  name: \"stage4_8/conv1\"\n  type: \"Convolution\"\n  bottom: \"stage4_7/sum\"\n  top: \"stage4_8/conv1\"\n  param {\n    lr_mult: 1.0\n    decay_mult: 1.0\n  }\n  convolution_param {\n    num_output: 32\n    pad: 0\n    kernel_size: 1\n    group: 1\n    stride: 1\n    weight_filler {\n      type: \"msra\"\n    }\n    dilation: 1\n  }\n}\nlayer {\n  name: \"stage4_8/conv1/relu\"\n  type: \"ReLU\"\n  bottom: \"stage4_8/conv1\"\n  top: \"stage4_8/conv1\"\n}\nlayer {\n  name: \"stage4_8/conv2\"\n  type: \"Convolution\"\n  bottom: \"stage4_8/conv1\"\n  top: \"stage4_8/conv2\"\n  param {\n    lr_mult: 1.0\n    decay_mult: 1.0\n  }\n  convolution_param {\n    num_output: 32\n    pad: 1\n    kernel_size: 3\n    group: 32\n    stride: 1\n    weight_filler {\n      type: \"msra\"\n    }\n    dilation: 1\n  }\n}\nlayer {\n  name: \"stage4_8/conv3\"\n  type: \"Convolution\"\n  bottom: \"stage4_8/conv2\"\n  top: \"stage4_8/conv3\"\n  param {\n    lr_mult: 1.0\n    decay_mult: 1.0\n  }\n  convolution_param {\n    num_output: 128\n    pad: 0\n    kernel_size: 1\n    group: 1\n    stride: 1\n    weight_filler {\n      type: \"msra\"\n    }\n    dilation: 1\n  }\n}\nlayer {\n  name: \"stage4_8/sum\"\n  type: \"Eltwise\"\n  bottom: \"stage4_7/sum\"\n  bottom: \"stage4_8/conv3\"\n  top: \"stage4_8/sum\"\n  eltwise_param {\n    operation: SUM\n  }\n}\nlayer {\n  name: \"stage4_8/relu\"\n  type: \"ReLU\"\n  bottom: \"stage4_8/sum\"\n  top: \"stage4_8/sum\"\n}\nlayer {\n  name: \"stage5_1/conv1\"\n  type: \"Convolution\"\n  bottom: \"stage4_8/sum\"\n  top: \"stage5_1/conv1\"\n  param {\n    lr_mult: 1.0\n    decay_mult: 1.0\n  }\n  convolution_param {\n    num_output: 32\n    pad: 0\n    kernel_size: 1\n    group: 1\n    stride: 1\n    weight_filler {\n      type: \"msra\"\n    }\n    dilation: 1\n  }\n}\nlayer {\n  name: \"stage5_1/conv1/relu\"\n  type: \"ReLU\"\n  bottom: \"stage5_1/conv1\"\n  top: \"stage5_1/conv1\"\n}\nlayer {\n  name: \"stage5_1/conv2\"\n  type: \"Convolution\"\n  bottom: \"stage5_1/conv1\"\n  top: \"stage5_1/conv2\"\n  param {\n    lr_mult: 1.0\n    decay_mult: 1.0\n  }\n  convolution_param {\n    num_output: 32\n    pad: 2\n    kernel_size: 3\n    group: 32\n    stride: 2\n    weight_filler {\n      type: \"msra\"\n    }\n    dilation: 2\n  }\n}\nlayer {\n  name: \"stage5_1/conv3\"\n  type: \"Convolution\"\n  bottom: \"stage5_1/conv2\"\n  top: \"stage5_1/conv3\"\n  param {\n    lr_mult: 1.0\n    decay_mult: 1.0\n  }\n  convolution_param {\n    num_output: 128\n    pad: 0\n    kernel_size: 1\n    group: 1\n    stride: 1\n    weight_filler {\n      type: \"msra\"\n    }\n    dilation: 1\n  }\n}\nlayer {\n  name: \"stage5_1/relu\"\n  type: \"ReLU\"\n  bottom: \"stage5_1/conv3\"\n  top: \"stage5_1/conv3\"\n}\nlayer {\n  name: \"stage5_2/conv1\"\n  type: \"Convolution\"\n  bottom: \"stage5_1/conv3\"\n  top: \"stage5_2/conv1\"\n  param {\n    lr_mult: 1.0\n    decay_mult: 1.0\n  }\n  convolution_param {\n    num_output: 32\n    pad: 0\n    kernel_size: 1\n    group: 1\n    stride: 1\n    weight_filler {\n      type: \"msra\"\n    }\n    dilation: 1\n  }\n}\nlayer {\n  name: \"stage5_2/conv1/relu\"\n  type: \"ReLU\"\n  bottom: \"stage5_2/conv1\"\n  top: \"stage5_2/conv1\"\n}\nlayer {\n  name: \"stage5_2/conv2\"\n  type: \"Convolution\"\n  bottom: \"stage5_2/conv1\"\n  top: \"stage5_2/conv2\"\n  param {\n    lr_mult: 1.0\n    decay_mult: 1.0\n  }\n  convolution_param {\n    num_output: 32\n    pad: 2\n    kernel_size: 3\n    group: 32\n    stride: 1\n    weight_filler {\n      type: \"msra\"\n    }\n    dilation: 2\n  }\n}\nlayer {\n  name: \"stage5_2/conv3\"\n  type: \"Convolution\"\n  bottom: \"stage5_2/conv2\"\n  top: \"stage5_2/conv3\"\n  param {\n    lr_mult: 1.0\n    decay_mult: 1.0\n  }\n  convolution_param {\n    num_output: 128\n    pad: 0\n    kernel_size: 1\n    group: 1\n    stride: 1\n    weight_filler {\n      type: \"msra\"\n    }\n    dilation: 1\n  }\n}\nlayer {\n  name: \"stage5_2/sum\"\n  type: \"Eltwise\"\n  bottom: \"stage5_1/conv3\"\n  bottom: \"stage5_2/conv3\"\n  top: \"stage5_2/sum\"\n  eltwise_param {\n    operation: SUM\n  }\n}\nlayer {\n  name: \"stage5_2/relu\"\n  type: \"ReLU\"\n  bottom: \"stage5_2/sum\"\n  top: \"stage5_2/sum\"\n}\nlayer {\n  name: \"stage5_3/conv1\"\n  type: \"Convolution\"\n  bottom: \"stage5_2/sum\"\n  top: \"stage5_3/conv1\"\n  param {\n    lr_mult: 1.0\n    decay_mult: 1.0\n  }\n  convolution_param {\n    num_output: 32\n    pad: 0\n    kernel_size: 1\n    group: 1\n    stride: 1\n    weight_filler {\n      type: \"msra\"\n    }\n    dilation: 1\n  }\n}\nlayer {\n  name: \"stage5_3/conv1/relu\"\n  type: \"ReLU\"\n  bottom: \"stage5_3/conv1\"\n  top: \"stage5_3/conv1\"\n}\nlayer {\n  name: \"stage5_3/conv2\"\n  type: \"Convolution\"\n  bottom: \"stage5_3/conv1\"\n  top: \"stage5_3/conv2\"\n  param {\n    lr_mult: 1.0\n    decay_mult: 1.0\n  }\n  convolution_param {\n    num_output: 32\n    pad: 2\n    kernel_size: 3\n    group: 32\n    stride: 1\n    weight_filler {\n      type: \"msra\"\n    }\n    dilation: 2\n  }\n}\nlayer {\n  name: \"stage5_3/conv3\"\n  type: \"Convolution\"\n  bottom: \"stage5_3/conv2\"\n  top: \"stage5_3/conv3\"\n  param {\n    lr_mult: 1.0\n    decay_mult: 1.0\n  }\n  convolution_param {\n    num_output: 128\n    pad: 0\n    kernel_size: 1\n    group: 1\n    stride: 1\n    weight_filler {\n      type: \"msra\"\n    }\n    dilation: 1\n  }\n}\nlayer {\n  name: \"stage5_3/sum\"\n  type: \"Eltwise\"\n  bottom: \"stage5_2/sum\"\n  bottom: \"stage5_3/conv3\"\n  top: \"stage5_3/sum\"\n  eltwise_param {\n    operation: SUM\n  }\n}\nlayer {\n  name: \"stage5_3/relu\"\n  type: \"ReLU\"\n  bottom: \"stage5_3/sum\"\n  top: \"stage5_3/sum\"\n}\nlayer {\n  name: \"stage5_4/conv1\"\n  type: \"Convolution\"\n  bottom: \"stage5_3/sum\"\n  top: \"stage5_4/conv1\"\n  param {\n    lr_mult: 1.0\n    decay_mult: 1.0\n  }\n  convolution_param {\n    num_output: 32\n    pad: 0\n    kernel_size: 1\n    group: 1\n    stride: 1\n    weight_filler {\n      type: \"msra\"\n    }\n    dilation: 1\n  }\n}\nlayer {\n  name: \"stage5_4/conv1/relu\"\n  type: \"ReLU\"\n  bottom: \"stage5_4/conv1\"\n  top: \"stage5_4/conv1\"\n}\nlayer {\n  name: \"stage5_4/conv2\"\n  type: \"Convolution\"\n  bottom: \"stage5_4/conv1\"\n  top: \"stage5_4/conv2\"\n  param {\n    lr_mult: 1.0\n    decay_mult: 1.0\n  }\n  convolution_param {\n    num_output: 32\n    pad: 2\n    kernel_size: 3\n    group: 32\n    stride: 1\n    weight_filler {\n      type: \"msra\"\n    }\n    dilation: 2\n  }\n}\nlayer {\n  name: \"stage5_4/conv3\"\n  type: \"Convolution\"\n  bottom: \"stage5_4/conv2\"\n  top: \"stage5_4/conv3\"\n  param {\n    lr_mult: 1.0\n    decay_mult: 1.0\n  }\n  convolution_param {\n    num_output: 128\n    pad: 0\n    kernel_size: 1\n    group: 1\n    stride: 1\n    weight_filler {\n      type: \"msra\"\n    }\n    dilation: 1\n  }\n}\nlayer {\n  name: \"stage5_4/sum\"\n  type: \"Eltwise\"\n  bottom: \"stage5_3/sum\"\n  bottom: \"stage5_4/conv3\"\n  top: \"stage5_4/sum\"\n  eltwise_param {\n    operation: SUM\n  }\n}\nlayer {\n  name: \"stage5_4/relu\"\n  type: \"ReLU\"\n  bottom: \"stage5_4/sum\"\n  top: \"stage5_4/sum\"\n}\nlayer {\n  name: \"stage6_1/conv4\"\n  type: \"Convolution\"\n  bottom: \"stage5_4/sum\"\n  top: \"stage6_1/conv4\"\n  param {\n    lr_mult: 1.0\n    decay_mult: 1.0\n  }\n  convolution_param {\n    num_output: 128\n    pad: 0\n    kernel_size: 1\n    group: 1\n    stride: 1\n    weight_filler {\n      type: \"msra\"\n    }\n    dilation: 1\n  }\n}\nlayer {\n  name: \"stage6_1/conv1\"\n  type: \"Convolution\"\n  bottom: \"stage5_4/sum\"\n  top: \"stage6_1/conv1\"\n  param {\n    lr_mult: 1.0\n    decay_mult: 1.0\n  }\n  convolution_param {\n    num_output: 32\n    pad: 0\n    kernel_size: 1\n    group: 1\n    stride: 1\n    weight_filler {\n      type: \"msra\"\n    }\n    dilation: 1\n  }\n}\nlayer {\n  name: \"stage6_1/conv1/relu\"\n  type: \"ReLU\"\n  bottom: \"stage6_1/conv1\"\n  top: \"stage6_1/conv1\"\n}\nlayer {\n  name: \"stage6_1/conv2\"\n  type: \"Convolution\"\n  bottom: \"stage6_1/conv1\"\n  top: \"stage6_1/conv2\"\n  param {\n    lr_mult: 1.0\n    decay_mult: 1.0\n  }\n  convolution_param {\n    num_output: 32\n    pad: 2\n    kernel_size: 3\n    group: 32\n    stride: 1\n    weight_filler {\n      type: \"msra\"\n    }\n    dilation: 2\n  }\n}\nlayer {\n  name: \"stage6_1/conv3\"\n  type: \"Convolution\"\n  bottom: \"stage6_1/conv2\"\n  top: \"stage6_1/conv3\"\n  param {\n    lr_mult: 1.0\n    decay_mult: 1.0\n  }\n  convolution_param {\n    num_output: 128\n    pad: 0\n    kernel_size: 1\n    group: 1\n    stride: 1\n    weight_filler {\n      type: \"msra\"\n    }\n    dilation: 1\n  }\n}\nlayer {\n  name: \"stage6_1/sum\"\n  type: \"Eltwise\"\n  bottom: \"stage6_1/conv4\"\n  bottom: \"stage6_1/conv3\"\n  top: \"stage6_1/sum\"\n  eltwise_param {\n    operation: SUM\n  }\n}\nlayer {\n  name: \"stage6_1/relu\"\n  type: \"ReLU\"\n  bottom: \"stage6_1/sum\"\n  top: \"stage6_1/sum\"\n}\nlayer {\n  name: \"stage6_2/conv1\"\n  type: \"Convolution\"\n  bottom: \"stage6_1/sum\"\n  top: \"stage6_2/conv1\"\n  param {\n    lr_mult: 1.0\n    decay_mult: 1.0\n  }\n  convolution_param {\n    num_output: 32\n    pad: 0\n    kernel_size: 1\n    group: 1\n    stride: 1\n    weight_filler {\n      type: \"msra\"\n    }\n    dilation: 1\n  }\n}\nlayer {\n  name: \"stage6_2/conv1/relu\"\n  type: \"ReLU\"\n  bottom: \"stage6_2/conv1\"\n  top: \"stage6_2/conv1\"\n}\nlayer {\n  name: \"stage6_2/conv2\"\n  type: \"Convolution\"\n  bottom: \"stage6_2/conv1\"\n  top: \"stage6_2/conv2\"\n  param {\n    lr_mult: 1.0\n    decay_mult: 1.0\n  }\n  convolution_param {\n    num_output: 32\n    pad: 2\n    kernel_size: 3\n    group: 32\n    stride: 1\n    weight_filler {\n      type: \"msra\"\n    }\n    dilation: 2\n  }\n}\nlayer {\n  name: \"stage6_2/conv3\"\n  type: \"Convolution\"\n  bottom: \"stage6_2/conv2\"\n  top: \"stage6_2/conv3\"\n  param {\n    lr_mult: 1.0\n    decay_mult: 1.0\n  }\n  convolution_param {\n    num_output: 128\n    pad: 0\n    kernel_size: 1\n    group: 1\n    stride: 1\n    weight_filler {\n      type: \"msra\"\n    }\n    dilation: 1\n  }\n}\nlayer {\n  name: \"stage6_2/sum\"\n  type: \"Eltwise\"\n  bottom: \"stage6_1/sum\"\n  bottom: \"stage6_2/conv3\"\n  top: \"stage6_2/sum\"\n  eltwise_param {\n    operation: SUM\n  }\n}\nlayer {\n  name: \"stage6_2/relu\"\n  type: \"ReLU\"\n  bottom: \"stage6_2/sum\"\n  top: \"stage6_2/sum\"\n}\nlayer {\n  name: \"stage7_1/conv4\"\n  type: \"Convolution\"\n  bottom: \"stage6_2/sum\"\n  top: \"stage7_1/conv4\"\n  param {\n    lr_mult: 1.0\n    decay_mult: 1.0\n  }\n  convolution_param {\n    num_output: 128\n    pad: 0\n    kernel_size: 1\n    group: 1\n    stride: 1\n    weight_filler {\n      type: \"msra\"\n    }\n    dilation: 1\n  }\n}\nlayer {\n  name: \"stage7_1/conv1\"\n  type: \"Convolution\"\n  bottom: \"stage6_2/sum\"\n  top: \"stage7_1/conv1\"\n  param {\n    lr_mult: 1.0\n    decay_mult: 1.0\n  }\n  convolution_param {\n    num_output: 32\n    pad: 0\n    kernel_size: 1\n    group: 1\n    stride: 1\n    weight_filler {\n      type: \"msra\"\n    }\n    dilation: 1\n  }\n}\nlayer {\n  name: \"stage7_1/conv1/relu\"\n  type: \"ReLU\"\n  bottom: \"stage7_1/conv1\"\n  top: \"stage7_1/conv1\"\n}\nlayer {\n  name: \"stage7_1/conv2\"\n  type: \"Convolution\"\n  bottom: \"stage7_1/conv1\"\n  top: \"stage7_1/conv2\"\n  param {\n    lr_mult: 1.0\n    decay_mult: 1.0\n  }\n  convolution_param {\n    num_output: 32\n    pad: 2\n    kernel_size: 3\n    group: 32\n    stride: 1\n    weight_filler {\n      type: \"msra\"\n    }\n    dilation: 2\n  }\n}\nlayer {\n  name: \"stage7_1/conv3\"\n  type: \"Convolution\"\n  bottom: \"stage7_1/conv2\"\n  top: \"stage7_1/conv3\"\n  param {\n    lr_mult: 1.0\n    decay_mult: 1.0\n  }\n  convolution_param {\n    num_output: 128\n    pad: 0\n    kernel_size: 1\n    group: 1\n    stride: 1\n    weight_filler {\n      type: \"msra\"\n    }\n    dilation: 1\n  }\n}\nlayer {\n  name: \"stage7_1/sum\"\n  type: \"Eltwise\"\n  bottom: \"stage7_1/conv4\"\n  bottom: \"stage7_1/conv3\"\n  top: \"stage7_1/sum\"\n  eltwise_param {\n    operation: SUM\n  }\n}\nlayer {\n  name: \"stage7_1/relu\"\n  type: \"ReLU\"\n  bottom: \"stage7_1/sum\"\n  top: \"stage7_1/sum\"\n}\nlayer {\n  name: \"stage7_2/conv1\"\n  type: \"Convolution\"\n  bottom: \"stage7_1/sum\"\n  top: \"stage7_2/conv1\"\n  param {\n    lr_mult: 1.0\n    decay_mult: 1.0\n  }\n  convolution_param {\n    num_output: 32\n    pad: 0\n    kernel_size: 1\n    group: 1\n    stride: 1\n    weight_filler {\n      type: \"msra\"\n    }\n    dilation: 1\n  }\n}\nlayer {\n  name: \"stage7_2/conv1/relu\"\n  type: \"ReLU\"\n  bottom: \"stage7_2/conv1\"\n  top: \"stage7_2/conv1\"\n}\nlayer {\n  name: \"stage7_2/conv2\"\n  type: \"Convolution\"\n  bottom: \"stage7_2/conv1\"\n  top: \"stage7_2/conv2\"\n  param {\n    lr_mult: 1.0\n    decay_mult: 1.0\n  }\n  convolution_param {\n    num_output: 32\n    pad: 2\n    kernel_size: 3\n    group: 32\n    stride: 1\n    weight_filler {\n      type: \"msra\"\n    }\n    dilation: 2\n  }\n}\nlayer {\n  name: \"stage7_2/conv3\"\n  type: \"Convolution\"\n  bottom: \"stage7_2/conv2\"\n  top: \"stage7_2/conv3\"\n  param {\n    lr_mult: 1.0\n    decay_mult: 1.0\n  }\n  convolution_param {\n    num_output: 128\n    pad: 0\n    kernel_size: 1\n    group: 1\n    stride: 1\n    weight_filler {\n      type: \"msra\"\n    }\n    dilation: 1\n  }\n}\nlayer {\n  name: \"stage7_2/sum\"\n  type: \"Eltwise\"\n  bottom: \"stage7_1/sum\"\n  bottom: \"stage7_2/conv3\"\n  top: \"stage7_2/sum\"\n  eltwise_param {\n    operation: SUM\n  }\n}\nlayer {\n  name: \"stage7_2/relu\"\n  type: \"ReLU\"\n  bottom: \"stage7_2/sum\"\n  top: \"stage7_2/sum\"\n}\nlayer {\n  name: \"stage8_1/conv4\"\n  type: \"Convolution\"\n  bottom: \"stage7_2/sum\"\n  top: \"stage8_1/conv4\"\n  param {\n    lr_mult: 1.0\n    decay_mult: 1.0\n  }\n  convolution_param {\n    num_output: 128\n    pad: 0\n    kernel_size: 1\n    group: 1\n    stride: 1\n    weight_filler {\n      type: \"msra\"\n    }\n    dilation: 1\n  }\n}\nlayer {\n  name: \"stage8_1/conv1\"\n  type: \"Convolution\"\n  bottom: \"stage7_2/sum\"\n  top: \"stage8_1/conv1\"\n  param {\n    lr_mult: 1.0\n    decay_mult: 1.0\n  }\n  convolution_param {\n    num_output: 32\n    pad: 0\n    kernel_size: 1\n    group: 1\n    stride: 1\n    weight_filler {\n      type: \"msra\"\n    }\n    dilation: 1\n  }\n}\nlayer {\n  name: \"stage8_1/conv1/relu\"\n  type: \"ReLU\"\n  bottom: \"stage8_1/conv1\"\n  top: \"stage8_1/conv1\"\n}\nlayer {\n  name: \"stage8_1/conv2\"\n  type: \"Convolution\"\n  bottom: \"stage8_1/conv1\"\n  top: \"stage8_1/conv2\"\n  param {\n    lr_mult: 1.0\n    decay_mult: 1.0\n  }\n  convolution_param {\n    num_output: 32\n    pad: 2\n    kernel_size: 3\n    group: 32\n    stride: 1\n    weight_filler {\n      type: \"msra\"\n    }\n    dilation: 2\n  }\n}\nlayer {\n  name: \"stage8_1/conv3\"\n  type: \"Convolution\"\n  bottom: \"stage8_1/conv2\"\n  top: \"stage8_1/conv3\"\n  param {\n    lr_mult: 1.0\n    decay_mult: 1.0\n  }\n  convolution_param {\n    num_output: 128\n    pad: 0\n    kernel_size: 1\n    group: 1\n    stride: 1\n    weight_filler {\n      type: \"msra\"\n    }\n    dilation: 1\n  }\n}\nlayer {\n  name: \"stage8_1/sum\"\n  type: \"Eltwise\"\n  bottom: \"stage8_1/conv4\"\n  bottom: \"stage8_1/conv3\"\n  top: \"stage8_1/sum\"\n  eltwise_param {\n    operation: SUM\n  }\n}\nlayer {\n  name: \"stage8_1/relu\"\n  type: \"ReLU\"\n  bottom: \"stage8_1/sum\"\n  top: \"stage8_1/sum\"\n}\nlayer {\n  name: \"stage8_2/conv1\"\n  type: \"Convolution\"\n  bottom: \"stage8_1/sum\"\n  top: \"stage8_2/conv1\"\n  param {\n    lr_mult: 1.0\n    decay_mult: 1.0\n  }\n  convolution_param {\n    num_output: 32\n    pad: 0\n    kernel_size: 1\n    group: 1\n    stride: 1\n    weight_filler {\n      type: \"msra\"\n    }\n    dilation: 1\n  }\n}\nlayer {\n  name: \"stage8_2/conv1/relu\"\n  type: \"ReLU\"\n  bottom: \"stage8_2/conv1\"\n  top: \"stage8_2/conv1\"\n}\nlayer {\n  name: \"stage8_2/conv2\"\n  type: \"Convolution\"\n  bottom: \"stage8_2/conv1\"\n  top: \"stage8_2/conv2\"\n  param {\n    lr_mult: 1.0\n    decay_mult: 1.0\n  }\n  convolution_param {\n    num_output: 32\n    pad: 2\n    kernel_size: 3\n    group: 32\n    stride: 1\n    weight_filler {\n      type: \"msra\"\n    }\n    dilation: 2\n  }\n}\nlayer {\n  name: \"stage8_2/conv3\"\n  type: \"Convolution\"\n  bottom: \"stage8_2/conv2\"\n  top: \"stage8_2/conv3\"\n  param {\n    lr_mult: 1.0\n    decay_mult: 1.0\n  }\n  convolution_param {\n    num_output: 128\n    pad: 0\n    kernel_size: 1\n    group: 1\n    stride: 1\n    weight_filler {\n      type: \"msra\"\n    }\n    dilation: 1\n  }\n}\nlayer {\n  name: \"stage8_2/sum\"\n  type: \"Eltwise\"\n  bottom: \"stage8_1/sum\"\n  bottom: \"stage8_2/conv3\"\n  top: \"stage8_2/sum\"\n  eltwise_param {\n    operation: SUM\n  }\n}\nlayer {\n  name: \"stage8_2/relu\"\n  type: \"ReLU\"\n  bottom: \"stage8_2/sum\"\n  top: \"stage8_2/sum\"\n}\nlayer {\n  name: \"cls1/conv\"\n  type: \"Convolution\"\n  bottom: \"stage4_8/sum\"\n  top: \"cls1/conv\"\n  param {\n    lr_mult: 1.0\n    decay_mult: 1.0\n  }\n  param {\n    lr_mult: 1.0\n    decay_mult: 0.0\n  }\n  convolution_param {\n    num_output: 12\n    bias_term: true\n    pad: 0\n    kernel_size: 1\n    group: 1\n    stride: 1\n    weight_filler {\n      type: \"msra\"\n    }\n    dilation: 1\n  }\n}\nlayer {\n  name: \"cls1/permute\"\n  type: \"Permute\"\n  bottom: \"cls1/conv\"\n  top: \"cls1/permute\"\n  permute_param {\n    order: 0\n    order: 2\n    order: 3\n    order: 1\n  }\n}\nlayer {\n  name: \"cls1/flatten\"\n  type: \"Flatten\"\n  bottom: \"cls1/permute\"\n  top: \"cls1/flatten\"\n  flatten_param {\n    axis: 1\n  }\n}\nlayer {\n  name: \"loc1/conv\"\n  type: \"Convolution\"\n  bottom: \"stage4_8/sum\"\n  top: \"loc1/conv\"\n  param {\n    lr_mult: 1.0\n    decay_mult: 1.0\n  }\n  param {\n    lr_mult: 1.0\n    decay_mult: 0.0\n  }\n  convolution_param {\n    num_output: 24\n    bias_term: true\n    pad: 0\n    kernel_size: 1\n    group: 1\n    stride: 1\n    weight_filler {\n      type: \"msra\"\n    }\n    dilation: 1\n  }\n}\nlayer {\n  name: \"loc1/permute\"\n  type: \"Permute\"\n  bottom: \"loc1/conv\"\n  top: \"loc1/permute\"\n  permute_param {\n    order: 0\n    order: 2\n    order: 3\n    order: 1\n  }\n}\nlayer {\n  name: \"loc1/flatten\"\n  type: \"Flatten\"\n  bottom: \"loc1/permute\"\n  top: \"loc1/flatten\"\n  flatten_param {\n    axis: 1\n  }\n}\nlayer {\n  name: \"stage4_8/sum/prior_box\"\n  type: \"PriorBox\"\n  bottom: \"stage4_8/sum\"\n  bottom: \"data\"\n  top: \"stage4_8/sum/prior_box\"\n  prior_box_param {\n    min_size: 50.0\n    max_size: 100.0\n    aspect_ratio: 2.0\n    aspect_ratio: 0.5\n    aspect_ratio: 3.0\n    aspect_ratio: 0.3333333432674408\n    flip: false\n    clip: false\n    variance: 0.10000000149011612\n    variance: 0.10000000149011612\n    variance: 0.20000000298023224\n    variance: 0.20000000298023224\n    step: 16.0\n  }\n}\nlayer {\n  name: \"cls2/conv\"\n  type: \"Convolution\"\n  bottom: \"stage5_4/sum\"\n  top: \"cls2/conv\"\n  param {\n    lr_mult: 1.0\n    decay_mult: 1.0\n  }\n  param {\n    lr_mult: 1.0\n    decay_mult: 0.0\n  }\n  convolution_param {\n    num_output: 12\n    bias_term: true\n    pad: 0\n    kernel_size: 1\n    group: 1\n    stride: 1\n    weight_filler {\n      type: \"msra\"\n    }\n    dilation: 1\n  }\n}\nlayer {\n  name: \"cls2/permute\"\n  type: \"Permute\"\n  bottom: \"cls2/conv\"\n  top: \"cls2/permute\"\n  permute_param {\n    order: 0\n    order: 2\n    order: 3\n    order: 1\n  }\n}\nlayer {\n  name: \"cls2/flatten\"\n  type: \"Flatten\"\n  bottom: \"cls2/permute\"\n  top: \"cls2/flatten\"\n  flatten_param {\n    axis: 1\n  }\n}\nlayer {\n  name: \"loc2/conv\"\n  type: \"Convolution\"\n  bottom: \"stage5_4/sum\"\n  top: \"loc2/conv\"\n  param {\n    lr_mult: 1.0\n    decay_mult: 1.0\n  }\n  param {\n    lr_mult: 1.0\n    decay_mult: 0.0\n  }\n  convolution_param {\n    num_output: 24\n    bias_term: true\n    pad: 0\n    kernel_size: 1\n    group: 1\n    stride: 1\n    weight_filler {\n      type: \"msra\"\n    }\n    dilation: 1\n  }\n}\nlayer {\n  name: \"loc2/permute\"\n  type: \"Permute\"\n  bottom: \"loc2/conv\"\n  top: \"loc2/permute\"\n  permute_param {\n    order: 0\n    order: 2\n    order: 3\n    order: 1\n  }\n}\nlayer {\n  name: \"loc2/flatten\"\n  type: \"Flatten\"\n  bottom: \"loc2/permute\"\n  top: \"loc2/flatten\"\n  flatten_param {\n    axis: 1\n  }\n}\nlayer {\n  name: \"stage5_4/sum/prior_box\"\n  type: \"PriorBox\"\n  bottom: \"stage5_4/sum\"\n  bottom: \"data\"\n  top: \"stage5_4/sum/prior_box\"\n  prior_box_param {\n    min_size: 100.0\n    max_size: 150.0\n    aspect_ratio: 2.0\n    aspect_ratio: 0.5\n    aspect_ratio: 3.0\n    aspect_ratio: 0.3333333432674408\n    flip: false\n    clip: false\n    variance: 0.10000000149011612\n    variance: 0.10000000149011612\n    variance: 0.20000000298023224\n    variance: 0.20000000298023224\n    step: 32.0\n  }\n}\nlayer {\n  name: \"cls3/conv\"\n  type: \"Convolution\"\n  bottom: \"stage6_2/sum\"\n  top: \"cls3/conv\"\n  param {\n    lr_mult: 1.0\n    decay_mult: 1.0\n  }\n  param {\n    lr_mult: 1.0\n    decay_mult: 0.0\n  }\n  convolution_param {\n    num_output: 12\n    bias_term: true\n    pad: 0\n    kernel_size: 1\n    group: 1\n    stride: 1\n    weight_filler {\n      type: \"msra\"\n    }\n    dilation: 1\n  }\n}\nlayer {\n  name: \"cls3/permute\"\n  type: \"Permute\"\n  bottom: \"cls3/conv\"\n  top: \"cls3/permute\"\n  permute_param {\n    order: 0\n    order: 2\n    order: 3\n    order: 1\n  }\n}\nlayer {\n  name: \"cls3/flatten\"\n  type: \"Flatten\"\n  bottom: \"cls3/permute\"\n  top: \"cls3/flatten\"\n  flatten_param {\n    axis: 1\n  }\n}\nlayer {\n  name: \"loc3/conv\"\n  type: \"Convolution\"\n  bottom: \"stage6_2/sum\"\n  top: \"loc3/conv\"\n  param {\n    lr_mult: 1.0\n    decay_mult: 1.0\n  }\n  param {\n    lr_mult: 1.0\n    decay_mult: 0.0\n  }\n  convolution_param {\n    num_output: 24\n    bias_term: true\n    pad: 0\n    kernel_size: 1\n    group: 1\n    stride: 1\n    weight_filler {\n      type: \"msra\"\n    }\n    dilation: 1\n  }\n}\nlayer {\n  name: \"loc3/permute\"\n  type: \"Permute\"\n  bottom: \"loc3/conv\"\n  top: \"loc3/permute\"\n  permute_param {\n    order: 0\n    order: 2\n    order: 3\n    order: 1\n  }\n}\nlayer {\n  name: \"loc3/flatten\"\n  type: \"Flatten\"\n  bottom: \"loc3/permute\"\n  top: \"loc3/flatten\"\n  flatten_param {\n    axis: 1\n  }\n}\nlayer {\n  name: \"stage6_2/sum/prior_box\"\n  type: \"PriorBox\"\n  bottom: \"stage6_2/sum\"\n  bottom: \"data\"\n  top: \"stage6_2/sum/prior_box\"\n  prior_box_param {\n    min_size: 150.0\n    max_size: 200.0\n    aspect_ratio: 2.0\n    aspect_ratio: 0.5\n    aspect_ratio: 3.0\n    aspect_ratio: 0.3333333432674408\n    flip: false\n    clip: false\n    variance: 0.10000000149011612\n    variance: 0.10000000149011612\n    variance: 0.20000000298023224\n    variance: 0.20000000298023224\n    step: 32.0\n  }\n}\nlayer {\n  name: \"cls4/conv\"\n  type: \"Convolution\"\n  bottom: \"stage7_2/sum\"\n  top: \"cls4/conv\"\n  param {\n    lr_mult: 1.0\n    decay_mult: 1.0\n  }\n  param {\n    lr_mult: 1.0\n    decay_mult: 0.0\n  }\n  convolution_param {\n    num_output: 12\n    bias_term: true\n    pad: 0\n    kernel_size: 1\n    group: 1\n    stride: 1\n    weight_filler {\n      type: \"msra\"\n    }\n    dilation: 1\n  }\n}\nlayer {\n  name: \"cls4/permute\"\n  type: \"Permute\"\n  bottom: \"cls4/conv\"\n  top: \"cls4/permute\"\n  permute_param {\n    order: 0\n    order: 2\n    order: 3\n    order: 1\n  }\n}\nlayer {\n  name: \"cls4/flatten\"\n  type: \"Flatten\"\n  bottom: \"cls4/permute\"\n  top: \"cls4/flatten\"\n  flatten_param {\n    axis: 1\n  }\n}\nlayer {\n  name: \"loc4/conv\"\n  type: \"Convolution\"\n  bottom: \"stage7_2/sum\"\n  top: \"loc4/conv\"\n  param {\n    lr_mult: 1.0\n    decay_mult: 1.0\n  }\n  param {\n    lr_mult: 1.0\n    decay_mult: 0.0\n  }\n  convolution_param {\n    num_output: 24\n    bias_term: true\n    pad: 0\n    kernel_size: 1\n    group: 1\n    stride: 1\n    weight_filler {\n      type: \"msra\"\n    }\n    dilation: 1\n  }\n}\nlayer {\n  name: \"loc4/permute\"\n  type: \"Permute\"\n  bottom: \"loc4/conv\"\n  top: \"loc4/permute\"\n  permute_param {\n    order: 0\n    order: 2\n    order: 3\n    order: 1\n  }\n}\nlayer {\n  name: \"loc4/flatten\"\n  type: \"Flatten\"\n  bottom: \"loc4/permute\"\n  top: \"loc4/flatten\"\n  flatten_param {\n    axis: 1\n  }\n}\nlayer {\n  name: \"stage7_2/sum/prior_box\"\n  type: \"PriorBox\"\n  bottom: \"stage7_2/sum\"\n  bottom: \"data\"\n  top: \"stage7_2/sum/prior_box\"\n  prior_box_param {\n    min_size: 200.0\n    max_size: 300.0\n    aspect_ratio: 2.0\n    aspect_ratio: 0.5\n    aspect_ratio: 3.0\n    aspect_ratio: 0.3333333432674408\n    flip: false\n    clip: false\n    variance: 0.10000000149011612\n    variance: 0.10000000149011612\n    variance: 0.20000000298023224\n    variance: 0.20000000298023224\n    step: 32.0\n  }\n}\nlayer {\n  name: \"cls5/conv\"\n  type: \"Convolution\"\n  bottom: \"stage8_2/sum\"\n  top: \"cls5/conv\"\n  param {\n    lr_mult: 1.0\n    decay_mult: 1.0\n  }\n  param {\n    lr_mult: 1.0\n    decay_mult: 0.0\n  }\n  convolution_param {\n    num_output: 12\n    bias_term: true\n    pad: 0\n    kernel_size: 1\n    group: 1\n    stride: 1\n    weight_filler {\n      type: \"msra\"\n    }\n    dilation: 1\n  }\n}\nlayer {\n  name: \"cls5/permute\"\n  type: \"Permute\"\n  bottom: \"cls5/conv\"\n  top: \"cls5/permute\"\n  permute_param {\n    order: 0\n    order: 2\n    order: 3\n    order: 1\n  }\n}\nlayer {\n  name: \"cls5/flatten\"\n  type: \"Flatten\"\n  bottom: \"cls5/permute\"\n  top: \"cls5/flatten\"\n  flatten_param {\n    axis: 1\n  }\n}\nlayer {\n  name: \"loc5/conv\"\n  type: \"Convolution\"\n  bottom: \"stage8_2/sum\"\n  top: \"loc5/conv\"\n  param {\n    lr_mult: 1.0\n    decay_mult: 1.0\n  }\n  param {\n    lr_mult: 1.0\n    decay_mult: 0.0\n  }\n  convolution_param {\n    num_output: 24\n    bias_term: true\n    pad: 0\n    kernel_size: 1\n    group: 1\n    stride: 1\n    weight_filler {\n      type: \"msra\"\n    }\n    dilation: 1\n  }\n}\nlayer {\n  name: \"loc5/permute\"\n  type: \"Permute\"\n  bottom: \"loc5/conv\"\n  top: \"loc5/permute\"\n  permute_param {\n    order: 0\n    order: 2\n    order: 3\n    order: 1\n  }\n}\nlayer {\n  name: \"loc5/flatten\"\n  type: \"Flatten\"\n  bottom: \"loc5/permute\"\n  top: \"loc5/flatten\"\n  flatten_param {\n    axis: 1\n  }\n}\nlayer {\n  name: \"stage8_2/sum/prior_box\"\n  type: \"PriorBox\"\n  bottom: \"stage8_2/sum\"\n  bottom: \"data\"\n  top: \"stage8_2/sum/prior_box\"\n  prior_box_param {\n    min_size: 300.0\n    max_size: 400.0\n    aspect_ratio: 2.0\n    aspect_ratio: 0.5\n    aspect_ratio: 3.0\n    aspect_ratio: 0.3333333432674408\n    flip: false\n    clip: false\n    variance: 0.10000000149011612\n    variance: 0.10000000149011612\n    variance: 0.20000000298023224\n    variance: 0.20000000298023224\n    step: 32.0\n  }\n}\nlayer {\n  name: \"mbox_conf\"\n  type: \"Concat\"\n  bottom: \"cls1/flatten\"\n  bottom: \"cls2/flatten\"\n  bottom: \"cls3/flatten\"\n  bottom: \"cls4/flatten\"\n  bottom: \"cls5/flatten\"\n  top: \"mbox_conf\"\n  concat_param {\n    axis: 1\n  }\n}\nlayer {\n  name: \"mbox_loc\"\n  type: \"Concat\"\n  bottom: \"loc1/flatten\"\n  bottom: \"loc2/flatten\"\n  bottom: \"loc3/flatten\"\n  bottom: \"loc4/flatten\"\n  bottom: \"loc5/flatten\"\n  top: \"mbox_loc\"\n  concat_param {\n    axis: 1\n  }\n}\nlayer {\n  name: \"mbox_priorbox\"\n  type: \"Concat\"\n  bottom: \"stage4_8/sum/prior_box\"\n  bottom: \"stage5_4/sum/prior_box\"\n  bottom: \"stage6_2/sum/prior_box\"\n  bottom: \"stage7_2/sum/prior_box\"\n  bottom: \"stage8_2/sum/prior_box\"\n  top: \"mbox_priorbox\"\n  concat_param {\n    axis: 2\n  }\n}\nlayer {\n  name: \"mbox_conf_reshape\"\n  type: \"Reshape\"\n  bottom: \"mbox_conf\"\n  top: \"mbox_conf_reshape\"\n  reshape_param {\n    shape {\n      dim: 0\n      dim: -1\n      dim: 2\n    }\n  }\n}\nlayer {\n  name: \"mbox_conf_softmax\"\n  type: \"Softmax\"\n  bottom: \"mbox_conf_reshape\"\n  top: \"mbox_conf_softmax\"\n  softmax_param {\n    axis: 2\n  }\n}\nlayer {\n  name: \"mbox_conf_flatten\"\n  type: \"Flatten\"\n  bottom: \"mbox_conf_softmax\"\n  top: \"mbox_conf_flatten\"\n  flatten_param {\n    axis: 1\n  }\n}\nlayer {\n  name: \"detection_output\"\n  type: \"DetectionOutput\"\n  bottom: \"mbox_loc\"\n  bottom: \"mbox_conf_flatten\"\n  bottom: \"mbox_priorbox\"\n  top: \"detection_output\"\n  detection_output_param {\n    num_classes: 2\n    share_location: true\n    background_label_id: 0\n    nms_param {\n      nms_threshold: 0.44999998807907104\n      top_k: 100\n    }\n    code_type: CENTER_SIZE\n    keep_top_k: 100\n    confidence_threshold: 0.20000000298023224\n  }\n}\n" ("ProtoTxt")] -> w1
    frame Disabled {
      w7 = path "C:/serenial/libraries/g-augmented-reality-toolkit/LabVIEW/third-party/wechat_qrcode" ("base path")
      # "Load from File - for development only"
      n2 = Build Path(base path=w7, name or relative path=path "detect.prototxt" ("Filepath")) -> (appended path=w4:path)
      n3 = Build Path(base path=w7, name or relative path=path "detect.caffemodel" ("Filepath")) -> (appended path=w6:path)
      n4 = Read from Binary File(10:-1 ("count (1)"), 11:w6) -> (2:w5:string)  [unwired: 4 in, 3 out]
      n5 = Read from Text File(file (use dialog)=w4) -> (text=w3:string)  [unwired: 3 in, 3 out]
    }
    frame Enabled {
      # "https://github.com/WeChatCV/opencv_3rdparty"
    }
  }
  "Model" <- w2
  "ProtoTxt" <- w1
